vi "Uim900Send wrapper.vi"(0 "dwDevIndex":u32, 1 "bAckEna":i32, 5 "dwCanNodeId":u32, 7 "pSendDate":string, 9 "len":i32, 11 "error in (no error)":errorcluster caption="错误输入（无错误）", 12 "pAckDate":string) -> (4 "function return":u32, 8 "pSendDate out":string, 14 "pAckDate out":string, 15 "error out":errorcluster caption="错误输出")   [LabVIEW 2016, in "UISimCanFunc_wrapper.lvlib"]
doc: "_declspec (dllexport) DWORD Uim900Send_wrapper(DWORD dwDevIndex, DWORD dwCanNodeId, char pSendDate[], int len, BOOL bAckEna, char pAckDate[]);"
uses:
  <userlib>/UISimCanFunc_wrapper/UISimCanFunc_wrapper.lvlib
  <userlib>/UISimCanFunc_wrapper/UISimCanFunc_wrapper.dll
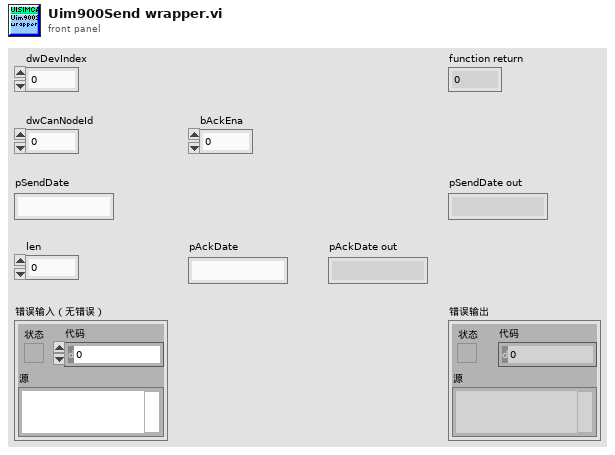
[diagram p1: front panel]
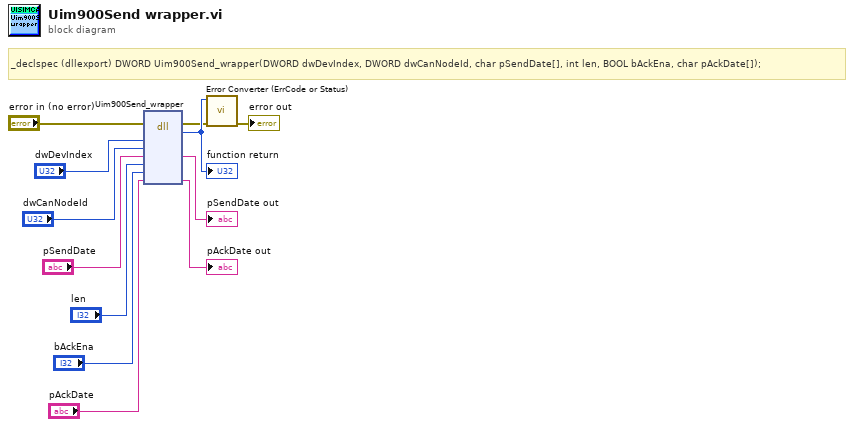
[diagram p0: block diagram]
diagram:
  # "_declspec (dllexport) DWORD Uim900Send_wrapper(DWORD dwDevIndex, DWORD dwCanNodeId, char pSendDate[], int len, BOOL bAckEna, char pAckDate[]);"
  n1 = dll-call lib="C:/Program Files (x86)/National Instruments/LabVIEW 2016/user.lib/UISimCanFunc_wrapper/UISimCanFunc_wrapper.*" fn="Uim900Send_wrapper"(error in="error in (no error)", "dwDevIndex"="dwDevIndex", "dwCanNodeId"="dwCanNodeId", "pSendDate"="pSendDate", "len"="len", "bAckEna"="bAckEna", "pAckDate"="pAckDate") -> (error out=w2:errorcluster, w12:u32, "pSendDate"=→"pSendDate out":string, "pAckDate"=→"pAckDate out":string)  [unwired: 6 in, 1 out]
  "function return" <- w12
  n2 = call <userlib>:"Error Converter (ErrCode or Status).vi"("error in (no error)"=w2, "error code"=w12) -> ("error out"=→"error out":errorcluster)  [unwired: 9 in]
